vi "URL to SL Tag Path.vi"(1 "URL":string) -> (0 "SL Tag Path":string)   [LabVIEW 2019, in "BNT_SLTools.lvlib"]
doc: "Convert CSPP URL to System Link Tag Path."
uses:
  <vilib>/Skyline/Utilities/Build Resource Name.vi
  BNT_SLTools.lvlib
  <vilib>/Skyline/Tag/Shared/NI Skyline Tag.lvlib
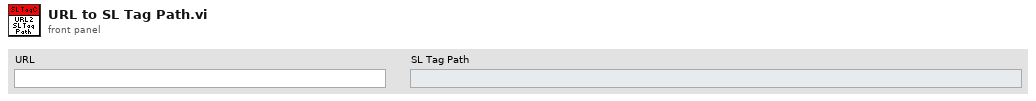
[diagram p1: front panel]
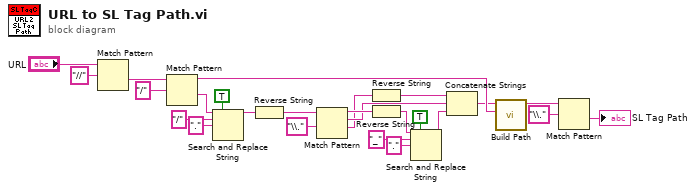
[diagram p0: block diagram]
diagram:
  n1 = Match Pattern(string="URL", regular expression="//") -> (after substring=w18:string)  [unwired: 1 in, 3 out]
  n2 = Match Pattern(string=w18, regular expression="/") -> (before substring=w17:string, after substring=w16:string)  [unwired: 1 in, 2 out]
  n3 = Search and Replace String(replace all?=TRUE ("replace all? (F)"), input string=w16, search string="/", replace string="." ("replace string (\"\")")) -> (result string=w20:string)  [unwired: 4 in, 3 out]
  n4 = Reverse String(1:w20) -> (0:w12:string)
  n5 = Match Pattern(string=w12, regular expression="\\.") -> (before substring=w11:string, match substring=w9:string, after substring=w8:string)  [unwired: 1 in, 1 out]
  n6 = Reverse String(1:w8) -> (0:w7:string)
  n7 = Reverse String(1:w11) -> (0:w3:string)
  n8 = Search and Replace String(replace all?=TRUE ("replace all? (F)"), input string=w3, search string="_", replace string="." ("replace string (\"\")")) -> (result string=w2:string)  [unwired: 4 in, 3 out]
  n9 = Concatenate Strings(w7, w9, w2) -> (w10:string)
  n10 = call <vilib>:"Build Path.vi"("namespace"=w17, "tag name"=w10) -> ("path"=w15:string)  [unwired: 9 in]
  n11 = Match Pattern(string=w15, regular expression="\\.") -> (after substring=→"SL Tag Path":string)  [unwired: 1 in, 3 out]
